vi "Basic SyRen 50 Controller.vi"() -> ()   [LabVIEW 2016]
uses:
  <vilib>/Instr/_visa.llb/VISA Configure Serial Port (Instr).vi
panel:
  in  "baud rate (9600)":u32=38400
  in  "VISA resource name":refnum<visa-resource-name>="COM1"
  in  "Seek Back Button":bool
  in  "Seek Forward Button":bool
  out "error out":errorcluster
  in  "Stop Button":bool
  in  "error in":errorcluster
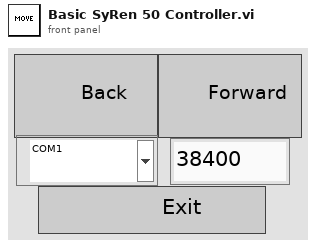
[diagram p1: front panel]
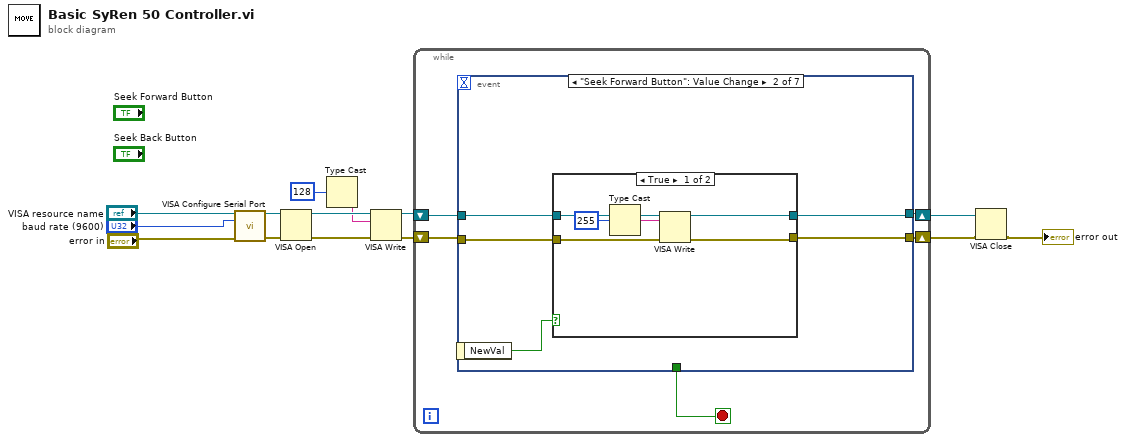
[diagram p0: block diagram]
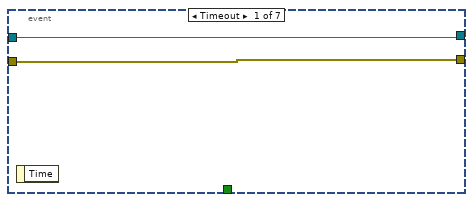
[diagram p2: hidden frame]
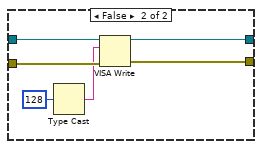
[diagram p3: hidden frame]
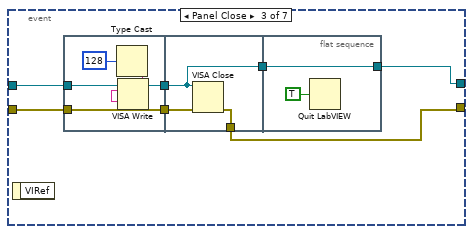
[diagram p4: hidden frame]
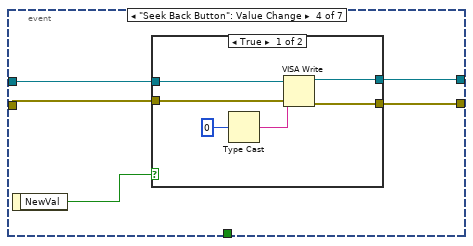
[diagram p5: hidden frame]
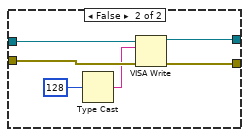
[diagram p6: hidden frame]
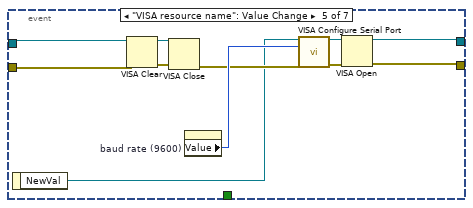
[diagram p7: hidden frame]
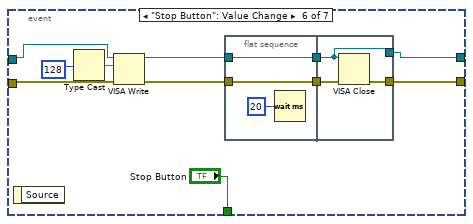
[diagram p8: hidden frame]
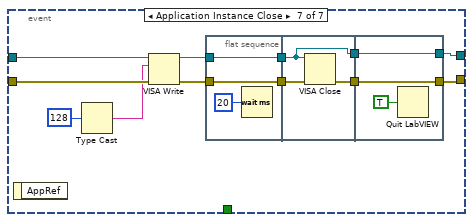
[diagram p9: hidden frame]
diagram:
  n1 = call-poly "VISA Configure Serial Port"("VISA resource name"="VISA resource name", "baud rate (9600)"="baud rate (9600)", "error in (no error)"="error in") -> ("VISA resource name out"=w12:refnum<visa-resource-name>, "error out"=w11:errorcluster)  [unwired: 11 in]
  n2 = VISA Open(error in (no error)=w11, VISA resource name=w12) -> (VISA resource name=w7:refnum<visa-resource-name>, error out=w8:errorcluster)  [unwired: 3 in]
  n3 = Type Cast(x=u8 128 ("Speed & Direction")) -> (*(type *) &x=w5:string)  [unwired: 1 in]
  n4 = VISA Write(VISA resource name=w7, write buffer=w5, error in (no error)=w8) -> (VISA resource name out=w4:refnum<visa-resource-name>, error out=w6:errorcluster)  [unwired: 1 out]
  n5 = while {
    shift-right: [w15] -> w1
    shift-left: w4 -> [w16]
    shift-right: [w18] -> w3
    shift-left: w6 -> [w19]
    stop <- w17 stop-if-true
    n6 = event shown="[1] \"Seek Forward Button\": Value Change" {
      selector: _ -> [_ _ _ _ _ _ _]
      dyn-events: _ -> [_ _ _ _ _ _ _]
      timeout: _ -> [_ _ _ _ _ _ _]
      tunnel: w19 -> [w21 w25 w45 w59 w75 w89 w107]
      tunnel: [w21 w26 w41 w60 w74 w92 w112] -> w18
      tunnel: [_ _ _ _ _ "Stop Button" _] -> w17
      tunnel: w16 -> [w20 w23 w43 w56 w76 w86 w105]
      tunnel: [w20 w22 w40 w57 w73 w84 w102] -> w15
      event Timeout {
        n7 = event-data() -> ()  [unwired: 1 in, 1 out]
      }
      event "Seek Forward Button": Value Change {
        n8 = event-data() -> ("NewVal"=w24:bool)  [unwired: 1 in]
        n9 = case shown="True" w24 {
          tunnel: [w30 w36] -> w26
          tunnel: w25 -> [w31 w37]
          tunnel: w23 -> [w28 w34]
          tunnel: [w27 w33] -> w22
          frame True {
            n10 = Type Cast(x=u8 255 ("Speed & Direction 2")) -> (*(type *) &x=w29:string)  [unwired: 1 in]
            n11 = VISA Write(VISA resource name=w28, write buffer=w29, error in (no error)=w31) -> (VISA resource name out=w27:refnum<visa-resource-name>, error out=w30:errorcluster)  [unwired: 1 out]
          }
          frame False {
            n12 = Type Cast(x=u8 128 ("Speed & Direction 2")) -> (*(type *) &x=w35:string)  [unwired: 1 in]
            n13 = VISA Write(VISA resource name=w34, write buffer=w35, error in (no error)=w37) -> (VISA resource name out=w33:refnum<visa-resource-name>, error out=w36:errorcluster)  [unwired: 1 out]
          }
        }
      }
      event Panel Close {
        n14 = event-data() -> ()  [unwired: 1 in, 1 out]
        n15 = flat-sequence {
          tunnel: w45 -> [w50]
          tunnel: [w50] -> w44
          tunnel: w43 -> [w48]
          tunnel: [w46] -> w42
          tunnel: w44 -> [w53]
          tunnel: w42 -> [w51]
          tunnel: [w52] -> w41
          tunnel: [w51] -> w39
          tunnel: [w54] -> w40
          tunnel: w39 -> [w54]
          frame #0 {
            n16 = Type Cast(x=u8 128 ("Speed & Direction")) -> (*(type *) &x=w47:string)  [unwired: 1 in]
            n17 = VISA Write(VISA resource name=w48, write buffer=w47) -> (VISA resource name out=w46:refnum<visa-resource-name>)  [unwired: 1 in, 2 out]
          }
          frame #1 {
            n18 = VISA Close(VISA resource name=w51, error in (no error)=w53) -> (error out=w52:errorcluster)
          }
          frame #2 {
            n19 = Quit LabVIEW(quit? (T)=TRUE) -> ()
          }
        }
      }
      event "Seek Back Button": Value Change {
        n20 = event-data() -> ("NewVal"=w58:bool)  [unwired: 1 in]
        n21 = case shown="True" w58 {
          tunnel: [w63 w70] -> w60
          tunnel: w59 -> [w64 w71]
          tunnel: [w62 w68] -> w57
          tunnel: w56 -> [w61 w67]
          frame True {
            n22 = Type Cast(x=u8 0 ("Speed & Direction 2")) -> (*(type *) &x=w65:string)  [unwired: 1 in]
            n23 = VISA Write(VISA resource name=w61, write buffer=w65, error in (no error)=w64) -> (VISA resource name out=w62:refnum<visa-resource-name>, error out=w63:errorcluster)  [unwired: 1 out]
          }
          frame False {
            n24 = Type Cast(x=u8 128 ("Speed & Direction 2")) -> (*(type *) &x=w69:string)  [unwired: 1 in]
            n25 = VISA Write(VISA resource name=w67, write buffer=w69, error in (no error)=w71) -> (VISA resource name out=w68:refnum<visa-resource-name>, error out=w70:errorcluster)  [unwired: 1 out]
          }
        }
      }
      event "VISA resource name": Value Change {
        n26 = event-data() -> ("NewVal"=w77:refnum<visa-resource-name>)  [unwired: 1 in]
        n27 = VISA Clear(VISA resource name=w76, error in (no error)=w75) -> (VISA resource name out=w79:refnum<visa-resource-name>, error out=w78:errorcluster)
        n28 = VISA Close(VISA resource name=w79, error in (no error)=w78) -> (error out=w82:errorcluster)
        n29 = property on="baud rate (9600)" class="DigNum (strict)"() -> ("Value"=w83:u32)  [unwired: 2 in, 2 out]
        n30 = call-poly "VISA Configure Serial Port"("VISA resource name"=w77, "baud rate (9600)"=w83, "error in (no error)"=w82) -> ("VISA resource name out"=w81:refnum<visa-resource-name>, "error out"=w80:errorcluster)  [unwired: 11 in]
        n31 = VISA Open(error in (no error)=w80, VISA resource name=w81) -> (VISA resource name=w73:refnum<visa-resource-name>, error out=w74:errorcluster)  [unwired: 3 in]
      }
      event "Stop Button": Value Change {
        n32 = event-data() -> ()  [unwired: 1 in, 1 out]
        n33 = Type Cast(x=i16 128 ("Speed & Direction")) -> (*(type *) &x=w87:string)  [unwired: 1 in]
        n34 = VISA Write(VISA resource name=w86, write buffer=w87, error in (no error)=w89) -> (VISA resource name out=w85:refnum<visa-resource-name>, error out=w88:errorcluster)  [unwired: 1 out]
        n35 = flat-sequence {
          tunnel: w88 -> [w96]
          tunnel: w85 -> [w97]
          tunnel: [w97] -> w91
          tunnel: [w96] -> w90
          tunnel: [w99] -> w92
          tunnel: w91 -> [w98]
          tunnel: w90 -> [w100]
          tunnel: [w98] -> w84
          frame #0 {
            n36 = Wait (ms)(milliseconds to wait=u32 20) -> ()  [unwired: 1 out]
          }
          frame #1 {
            n37 = VISA Close(VISA resource name=w98, error in (no error)=w100) -> (error out=w99:errorcluster)
          }
        }
      }
      event Application Instance Close {
        n38 = event-data() -> ()  [unwired: 1 in, 1 out]
        n39 = Type Cast(x=i16 128 ("Speed & Direction")) -> (*(type *) &x=w103:string)  [unwired: 1 in]
        n40 = VISA Write(VISA resource name=w105, write buffer=w103, error in (no error)=w107) -> (VISA resource name out=w104:refnum<visa-resource-name>, error out=w106:errorcluster)  [unwired: 1 out]
        n41 = flat-sequence {
          tunnel: w106 -> [w114]
          tunnel: w104 -> [w115]
          tunnel: [w115] -> w110
          tunnel: [w114] -> w109
          tunnel: w110 -> [w116]
          tunnel: w109 -> [w118]
          tunnel: [w117] -> w108
          tunnel: [w116] -> w101
          tunnel: [w121] -> w112
          tunnel: w108 -> [w121]
          tunnel: [w119] -> w102
          tunnel: w101 -> [w119]
          frame #0 {
            n42 = Wait (ms)(milliseconds to wait=u32 20) -> ()  [unwired: 1 out]
          }
          frame #1 {
            n43 = VISA Close(VISA resource name=w116, error in (no error)=w118) -> (error out=w117:errorcluster)
          }
          frame #2 {
            n44 = Quit LabVIEW(quit? (T)=TRUE) -> ()
          }
        }
      }
    }
  }
  n45 = VISA Close(VISA resource name=w1, error in (no error)=w3) -> (error out=→"error out":errorcluster)
